vi "Read Outputs to system.vi"(8 "error in":errorcluster, 11 "AppStateMachine runtime in":refnum<class "AppStateMachine runtime.lvclass">) -> (0 "error out":errorcluster, 2 "Outputs to system":T1, 3 "AppStateMachine runtime out":refnum<class "AppStateMachine runtime.lvclass">)   [LabVIEW 2017, in "AppStateMachine runtime.lvclass"]
uses:
  AppStateMachine runtime.lvclass
  configuration/output data indices.ctl
  AppStateMachine runtime.lvclass/AppStateMachine runtime.ctl
  configuration/AppStateMachine configuration.lvclass
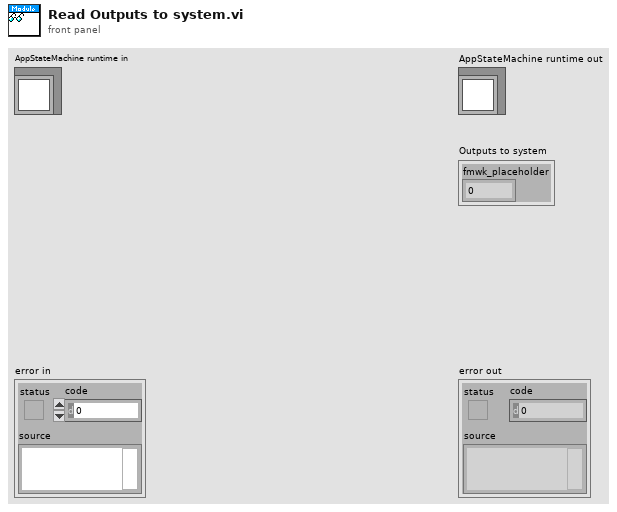
[diagram p1: front panel]
types:
  T1 = typedef "AppStateMachine configuration.lvclass/output data indices.ctl" = cluster{"fmwk_placeholder":i32}
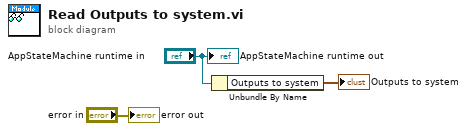
[diagram p0: block diagram]
diagram:
  n1 = Unbundle By Name("AppStateMachine runtime in") -> ("Outputs to system"=→"Outputs to system":T1)
  "error out" <- "error in"
  "AppStateMachine runtime out" <- "AppStateMachine runtime in"
